vi "add_one.vi"(10 "Numeric":dbl) -> (2 "x+1":dbl)   [LabVIEW 2021, in "Child.lvclass"]
uses:
  Child.lvclass
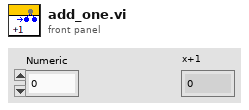
[diagram p1: front panel]
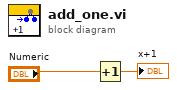
[diagram p0: block diagram]
diagram:
  n1 = Increment(x="Numeric") -> (x+1=→"x+1":dbl)
